vi "Global ADCarray.vi"() -> ()   [LabVIEW 2014]
panel:
  out "Waveform Array-FFT":waveform(dbl)[](array[waveform])
  in  "Array - FFT":i32[][](array[numeric])
  in  "Array - Fit":i32[][](array[numeric])
  in  "FCH7":i32[](array[numeric])
  in  "FCH6":i32[](array[numeric])
  in  "FCH5":i32[](array[numeric])
  in  "FCH4":i32[](array[numeric])
  in  "FCH3":i32[](array[numeric])
  in  "FCH2":i32[](array[numeric])
  in  "FCH1":i32[](array[numeric])
  in  "FCH0":i32[](array[numeric])
  out "Waveform Array-Fitting":waveform(dbl)[](array[waveform])
  in  "Nb pixel":i32
  out "ADC array":i32[][](array[numeric])
  in  "CH7":i32[](array[numeric])
  in  "CH6":i32[](array[numeric])
  in  "CH5":i32[](array[numeric])
  in  "CH4":i32[](array[numeric])
  in  "CH3":i32[](array[numeric])
  in  "CH2":i32[](array[numeric])
  in  "CH1":i32[](array[numeric])
  in  "CH0":i32[](array[numeric])
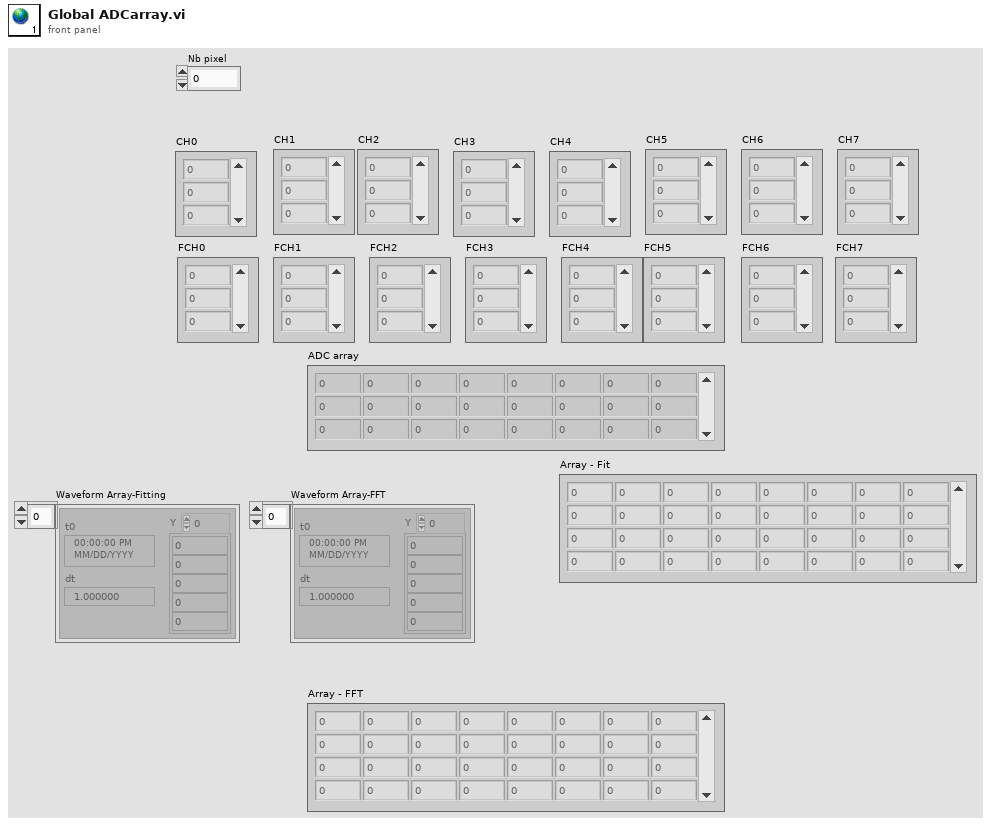
[diagram p1: front panel]
diagram:
